vi "Configure Trigger (Auto Trigger).vi"(0 "VISA resource name":refnum<visa-resource-name>, 5 "Timeout Value (100E-3 s)":dbl=0.1, 7 "Enable Auto Trigger (F: Disable)":bool, 11 "error in (no error)":errorcluster) -> (4 "VISA resource name out":refnum<visa-resource-name>, 15 "error out":errorcluster)   [LabVIEW 2018, in "Agilent MXA Series.lvlib"]
doc: "Sets the time that the analyzer will wait for the trigger conditions to be met. If they are not met after that much time, then the analyzer is triggered anyway."
uses:
  Agilent MXA Series.lvlib
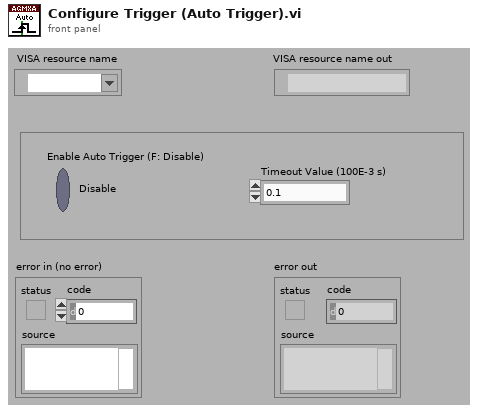
[diagram p1: front panel]
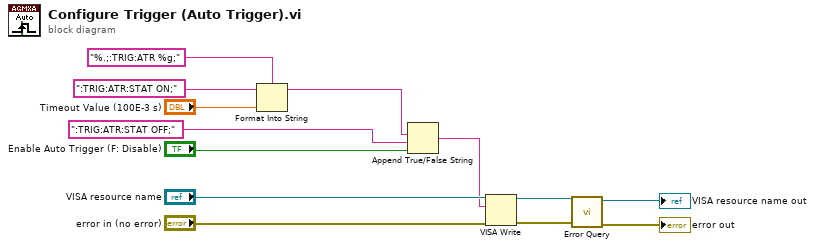
[diagram p0: block diagram]
diagram:
  n1 = Format Into String(format string="%.;:TRIG:ATR %g;", initial string=":TRIG:ATR:STAT ON;" ("format string"), "Timeout Value (100E-3 s)") -> (resulting string=w10:string)  [unwired: 1 in, 1 out]
  n2 = Append True/False String(1:"Enable Auto Trigger (F: Disable)", 2:":TRIG:ATR:STAT OFF;" ("false string"), 3:w10) -> (0:w1:string)  [unwired: 1 in]
  n3 = VISA Write(VISA resource name="VISA resource name", write buffer=w1, error in (no error)="error in (no error)") -> (VISA resource name out=w4:refnum<visa-resource-name>, error out=w5:errorcluster)  [unwired: 1 out]
  n4 = call "Error Query.vi"("error in (no error)"=w5, "VISA resource name"=w4) -> ("error out"=→"error out":errorcluster, "VISA resource name out"=→"VISA resource name out":refnum<visa-resource-name>)  [unwired: 6 in, 2 out]
